vi "Format Max P Stabil data for plot.vi"(11 "Data Array":dbl[][](array[numeric])) -> (3 "JV Curve":cluster{"Y":dbl[], "Y":dbl[]}[](graph))   [LabVIEW 2011]
panel:
  in  "Tab Control 4":enum32{"Page 1"}(tab)
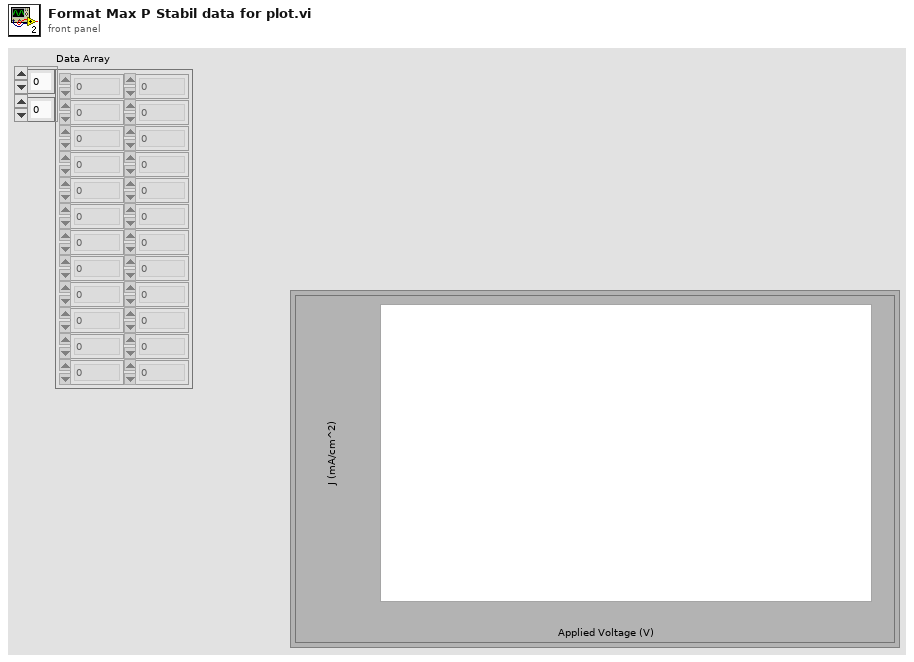
[diagram p1: front panel]
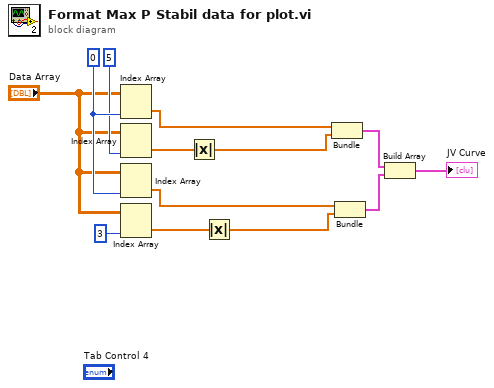
[diagram p0: block diagram]
diagram:
  w8 = 0
  n1 = Index Array(array="Data Array", index (col)=w8) -> (element=w13:dbl[])  [unwired: 1 in]
  n2 = Index Array(array="Data Array", index (col)=5) -> (element=w2:dbl[])  [unwired: 1 in]
  n3 = Index Array(array="Data Array", index (col)=w8) -> (element=w12:dbl[])  [unwired: 1 in]
  n4 = Index Array(array="Data Array", index (col)=3 ("disabled index (col)")) -> (element=w4:dbl[])  [unwired: 1 in]
  n5 = Absolute Value(x=w2) -> (abs(x)=w1:dbl[])
  n6 = Absolute Value(x=w4) -> (abs(x)=w3:dbl[])
  n7 = Bundle("Data Array"=w13, w1) -> (w10:cluster{"Data Array":dbl[], dbl[]})  [unwired: 1 in]
  n8 = Bundle("Data Array"=w12, w3) -> (w11:cluster{"Data Array":dbl[], dbl[]})  [unwired: 1 in]
  n9 = Build Array(w10, w11) -> (→"JV Curve":cluster{"Data Array":dbl[], dbl[]}[])
